vi "LVClass_CorrectionDataManager GetGeneralSetUp.vi"(0 "CorrectionDataManager in":refnum<class "CorrectionDataManager.lvclass">, 11 "error in (no error)":errorcluster) -> (4 "CorrectionDataManager out":refnum<class "CorrectionDataManager.lvclass">, 8 "general":T1, 15 "error out":errorcluster)   [LabVIEW 2020, in "CorrectionDataManager.lvclass"]
doc: "Haso and Wavefront corrector specifications getter.\n\n<B>corrdata_managerIn</B> : CorrDataManager object.\n<B>corrdata_managerOut</B> : CorrDataManager object.\n<B>nb_actuators</B> : Wavefront corrector actuators count.\n<B>wavefrontcorrector_name</B> : Wavefront corrector pretty name.\n<B>wavefrontcorrector_serial_number</B> : Wavefront corrector serial number.\n<B>haso_slopes_size</B> : Haso measures (HasoSlopes) dimensions.\n<B>haso_slopes_step</B> : Haso measures (HasoSlopes) sampling step (um).\n<B>haso_serial_number</B> : Haso serial number."
uses:
  CorrectionDataManager.lvclass
  CasaoManagerGeneralSpecifications.ctl
  General dimensions definition.ctl
  Point2D.ctl
  Point2Df.ctl
  CorrectionDataManager.lvclass/CorrectionDataManager.ctl
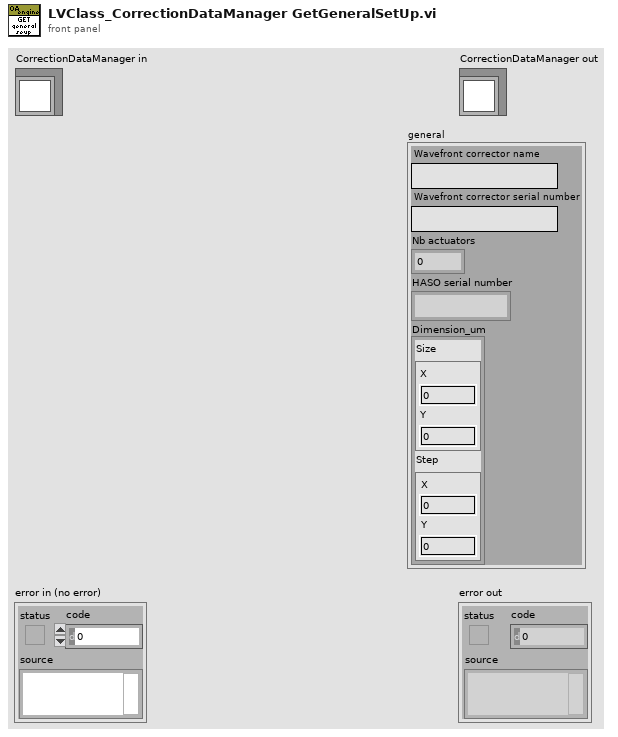
[diagram p1: front panel]
types:
  T1 = typedef "CasaoManagerGeneralSpecifications.ctl" = cluster{"Wavefront corrector name":string, "Wavefront corrector serial number":string, "Nb actuators":i32, "HASO serial number":string, "Dimension_um":T2}
  T2 = typedef "General dimensions definition.ctl" = cluster{"Size":T3, "Step":T4}
  T3 = typedef "Point2D.ctl" = cluster{"X":u32, "Y":u32}
  T4 = typedef "Point2Df.ctl" = cluster{"X":sgl, "Y":sgl}
  T5 = typedef "ClassID.ctl" = i64
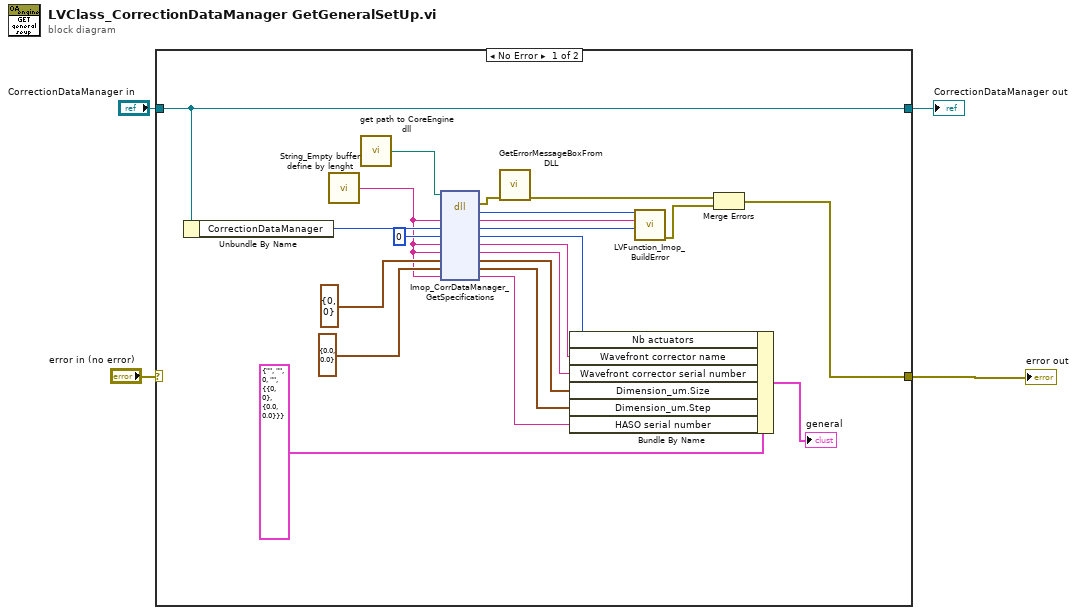
[diagram p0: block diagram]
diagram:
  n1 = case shown="No Error" "error in (no error)" {
    selector: "error in (no error)" -> [_ w28]
    tunnel: [w20 w28] -> w2
    tunnel: [w19 w27] -> w1
    tunnel: "CorrectionDataManager in" -> [w19 w27]
    frame No Error {
      n2 = Unbundle By Name(w19) -> ("CorrectionDataManager"=w18:T5)
      n3 = call "String_Empty buffer define by lenght.vi"() -> ("Empty buffer"=w6:string)  [unwired: 1 in]
      n4 = call "get path to CoreEngine dll.vi"() -> ("path to wavekit library"=w24:path)  [unwired: 14 in, 1 out]
      n5 = dll-call lib="D:/soft/HASO_v3/SVN_trunk/ImOpCoreEngine4_LV2011/DLLs/c_interface_vc100.dll" fn="Imop_CorrDataManager_GetSpecifications"(path in=w24, "message"=w6, "WavefrontCorrection"=w18, "Nb actuators"=0, "arg4"=w6, "arg5"=w6, "arg6"=T3 {"X"=0, "Y"=0} ("Size1"), "arg7"=T4 {"X"=0.0, "Y"=0.0} ("Step"), "arg8"=w6) -> (error out=w23:errorcluster, "return type"=w26:i32, "message"=w25:string, "WavefrontCorrection"=w5:i64, "Nb actuators"=w7:i32, "arg4"=w8:string, "arg5"=w9:string, "arg6"=w12:T3, "arg7"=w11:T4, "arg8"=w10:string)  [unwired: 2 in, 1 out]
      n6 = call "GetErrorMessageBoxFromDLL.vi"("error IN"=w23) -> ("error OUT"=w22:errorcluster)  [unwired: 10 in]
      n7 = Bundle By Name(cluster=T1 {"Wavefront corrector name"="", "Wavefront corrector serial number"="", "Nb actuators"=0, "HASO serial number"="", "Dimension_um"={"Size"={"X"=0, "Y"=0}, "Step"={"X"=0.0, "Y"=0.0}}} ("Nb actuators"), "Nb actuators"=w7, "Wavefront corrector name"=w8, "Wavefront corrector serial number"=w9, "Dimension_um.Size"=w12, "Dimension_um.Step"=w11, "HASO serial number"=w10) -> (→"general":T1)
      n8 = call "LVFunction_Imop_BuildError.vi"("code"=w26, "String to Prepend to source (\"\")"=w25, "Adresse"=w5) -> ("error out"=w21:errorcluster)  [unwired: 12 in]
      n9 = Merge Errors(w22, w21) -> (w20:errorcluster)
    }
    frame Error {
    }
  }
  "error out" <- w2
  "CorrectionDataManager out" <- w1
